vi "set_request_body.vi"(8 "error in":errorcluster, 10 "body":string, 11 "obj in":refnum<class "RequestBuilder.lvclass">) -> (0 "error out":errorcluster, 2 "success":bool, 3 "obj out":refnum<class "RequestBuilder.lvclass">)   [LabVIEW 2020, in "reqwest.lvlib" / "RequestBuilder.lvclass"]
doc: "Use this when you need to send raw text, XML data, binary files, or any custom content format that the other methods don't handle - it does NOT set any headers automatically, so you must manually set the appropriate Content-Type header using request_builder_header."
uses:
  RequestBuilder.lvclass
  RequestBuilder.lvclass/RequestBuilder.ctl
  lv_reqwest_64.so
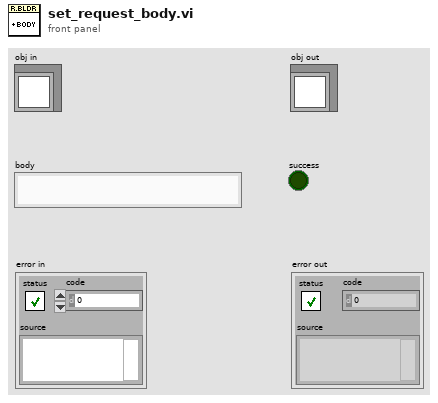
[diagram p1: front panel]
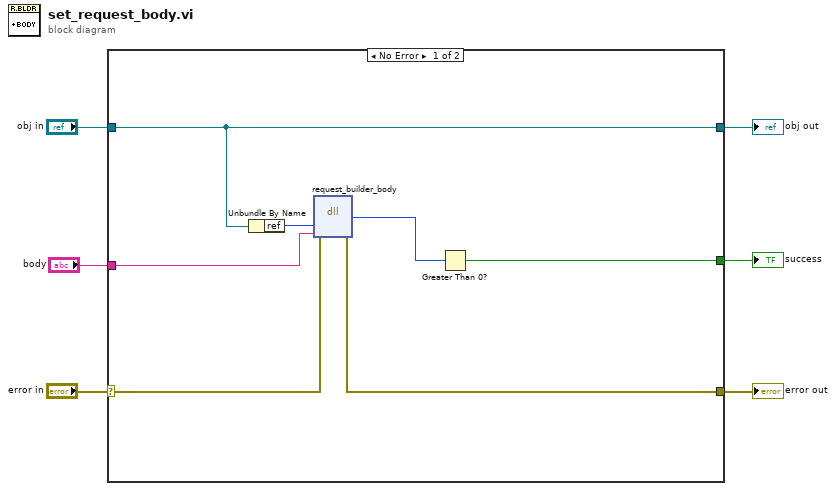
[diagram p0: block diagram]
diagram:
  n1 = case shown="No Error" "error in" {
    selector: "error in" -> [w13 w15]
    tunnel: "obj in" -> [w12 w14]
    tunnel: [w7 w15] -> w4
    tunnel: [w12 w14] -> w3
    tunnel: "body" -> [w10 _]
    tunnel: [w8 _] -> w1
    frame No Error {
      n2 = Unbundle By Name(w12) -> ("ref"=w11:u64)
      n3 = dll-call lib="home/jim-kring/Projects/reqwest-rs-labview/lv_src/lv_reqwest_*.*" fn="request_builder_body"(error in=w13, "builder_ptr"=w11, "body"=w10) -> (error out=w7:errorcluster, "Return Value"=w9:u8)  [unwired: 4 in, 1 out]
      n4 = Greater Than 0?(x=w9) -> (x > 0?=w8:bool)
    }
    frame Error {
    }
  }
  "error out" <- w4
  "obj out" <- w3
  "success" <- w1
